vi "Write to Active Logs.vi"(7 "Async Data in":T1, 8 "error in (no error)":errorcluster, 10 "Data in":dbl[](array[numeric]), 11 "Waveform Receive in":refnum<class "Waveform Receive.lvclass">) -> (0 "error out":errorcluster, 2 "Data out":dbl[](array[numeric]), 3 "Waveform Receive out":refnum<class "Waveform Receive.lvclass">)   [LabVIEW 2015, in "Waveform Data Logger Engine.lvlib" / "Waveform Receive.lvclass"]
uses:
  Waveform Receive.lvclass
  Types/Async Data.ctl
  <vilib>/NI VeriStand/Custom Device Waveform API/Multiple Waveforms Read (DBL)/Multiple Waveforms Read (DBL).lvclass
  Utilities/Reference Dictionary/Reference Dictionary.lvclass
  Types/Wfm Acq Data.ctl
  Waveform Log/Waveform Log.lvclass
  Types/Async Communication.ctl
  Types/Check File Loop Cmd.ctl
  Waveform Receive.lvclass/Waveform Receive.ctl
  Waveform Log/Waveform Log.lvclass/Waveform Log.ctl
  Logs/Segmented Logs/Segmented Log/Segmented Log.lvclass/Segmented Log.ctl
  Shared/Classes/Log File Specifications/Log File Specification/Log File Specification.lvclass/Log File Specification.ctl
  Shared/Classes/Log File Specifications/Waveform TDMS Log File Specification/Waveform TDMS Log File Specification.lvclass/Waveform TDMS Log File Specification.ctl
  Logs/Log Files/Log File/Log File.lvclass/Log File.ctl
  Logs/Log Files/TDMS Log File/TDMS Log File.lvclass/TDMS Log File.ctl
  Logs/Log Files/Text Log File/Text Log File.lvclass/Text Log File.ctl
  Logs/Segmented Logs/Footprint Segmented Log/Footprint Segmented Log.lvclass/Footprint Segmented Log.ctl
  Logs/Segmented Logs/Time Segmented Log/Time Segmented Log.lvclass/Time Segmented Log.ctl
  Waveform Log/Get Waveform In Range.vi
  Waveform Log/Write to Waveform Log Instance.vi
  Waveform Log/Update Log Status.vi
  Logs/Segmented Logs/Segmented Log/Write Waveform to Log File Instance.vi
  Shared/Classes/Log File Specifications/Log File Specification/Get Log Specification Type.vi
  Shared/Classes/Log File Specifications/Waveform TDMS Log File Specification/Get Current Group.vi
  Logs/Log Files/Log File/Get Log File Type.vi
  Logs/Log Files/Log File/Write Channel to Log File.vi
  Logs/Log Files/TDMS Log File/Set TDMS Channel Property.vi
  Logs/Log Files/TDMS Log File/Copy Channel Properties.vi
  Logs/Segmented Logs/Segmented Log/Check Close File.vi
  Logs/Segmented Logs/Segmented Log/Check Open File.vi
  Logs/Log Files/TDMS Log File/Write Channel to TDMS Log File.vi
  Logs/Log Files/Text Log File/Write Channel to Text Log File.vi
  Logs/Segmented Logs/Segmented Log/Close Log File Instance.vi
  Logs/Segmented Logs/Segmented Log/Segment Log File.vi
  Logs/Segmented Logs/Segmented Log/Open Log File Instance.vi
  Logs/Log Files/Log File/Close Log File.vi
  Logs/Segmented Logs/Segmented Log/Make File Read-Only.vi
  Logs/Segmented Logs/Segmented Log/On Segmented Log Complete.vi
  Logs/Segmented Logs/Segmented Log/On File Close.vi
  Logs/Segmented Logs/Footprint Segmented Log/Segment Log File (Footprint).vi
  Logs/Segmented Logs/Time Segmented Log/Segment Log File (Time).vi
  Shared/Classes/Log File Specifications/Log File Specification/Open Log File.vi
  Shared/Classes/Log File Specifications/Log File Specification/Set Path Tag.vi
  Logs/Segmented Logs/Segmented Log/On File Open.vi
  Shared/Classes/Log File Specifications/Log File Specification/Set Filename Offset.vi
  Logs/Log Files/TDMS Log File/Close TDMS Log File.vi
  Logs/Log Files/Text Log File/Close Text Log File.vi
  Logs/Segmented Logs/Segmented Log/Get Current Log File Instance.vi
  Logs/Log Files/Log File/Get File Size.vi
  Logs/Log Files/Log File/Get Start Time.vi
  Shared/Classes/Log File Specifications/Log File Specification/Build File Path.vi
  Shared/Classes/Log File Specifications/Log File Specification/Resolve File Conflicts.vi
  Waveform Log/Check Instance Done.vi
  <vilib>/Utility/error.llb/Error Cluster From Error Code.vi
  Shared/Classes/Log File Specifications/Log File Specification/Initialize Log File.vi
  <vilib>/Utility/libraryn.llb/Create Directory Recursive.vi
  <vilib>/Utility/libraryn.llb/Check if File or Folder Exists.vi
  <vilib>/Utility/libraryn.llb/Get File Extension.vi
  Logs/Log Files/Text Log File/Text Log File.lvclass
  Logs/Log Files/TDMS Log File/TDMS Log File.lvclass
  Logs/Log Files/Log File/Log File.lvclass
  Logs/Segmented Logs/Time Segmented Log/Time Segmented Log.lvclass
  Logs/Segmented Logs/Footprint Segmented Log/Footprint Segmented Log.lvclass
  Shared/Classes/Log File Specifications/Waveform TDMS Log File Specification/Waveform TDMS Log File Specification.lvclass
  Waveform Data Logger Engine.lvlib
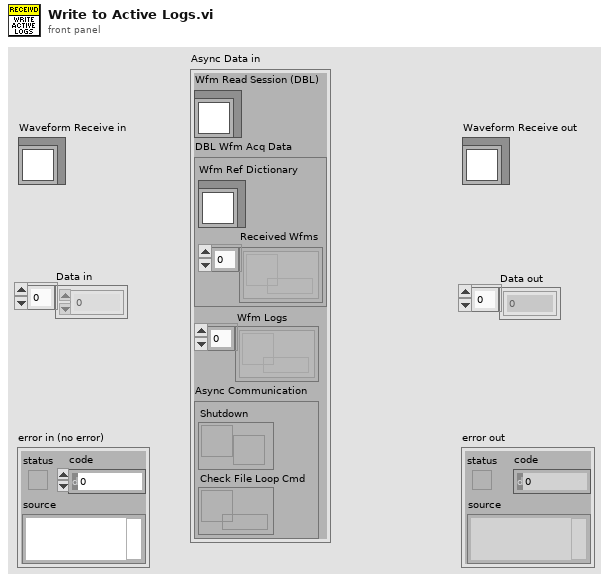
[diagram p1: front panel]
types:
  T1 = typedef "Waveform Data Logger Engine.lvlib/Async Data.ctl" = cluster{"Wfm Read Session (DBL)":refnum<class "Multiple Waveforms Read (DBL).lvclass">, "DBL Wfm Acq Data":T2, "Wfm Logs":refnum<data-value>[], "Async Communication":T3}
  T2 = typedef "Waveform Data Logger Engine.lvlib/Wfm Acq Data.ctl" = cluster{"Wfm Ref Dictionary":refnum<class "Reference Dictionary.lvclass">, "Received Wfms":refnum<data-value>[]}
  T3 = typedef "Waveform Data Logger Engine.lvlib/Async Communication.ctl" = cluster{"Shutdown":refnum<user-event>, "Check File Loop Cmd":refnum<queue>}
  T4 = typedef "Waveform Data Logger Engine.lvlib/Waveform Receive.lvclass/Associated Log.ctl" = cluster{"Log Index":i32, "Wfm Index":i32}
  T5 = typedef "Waveform Data Logger Engine.lvlib/Waveform Receive.lvclass/Wfm Info.ctl" = cluster{"Segment ID":u64, "Size":i32, "dt":dbl, "t0":timestamp, "offset":u64, "receive time":timestamp}
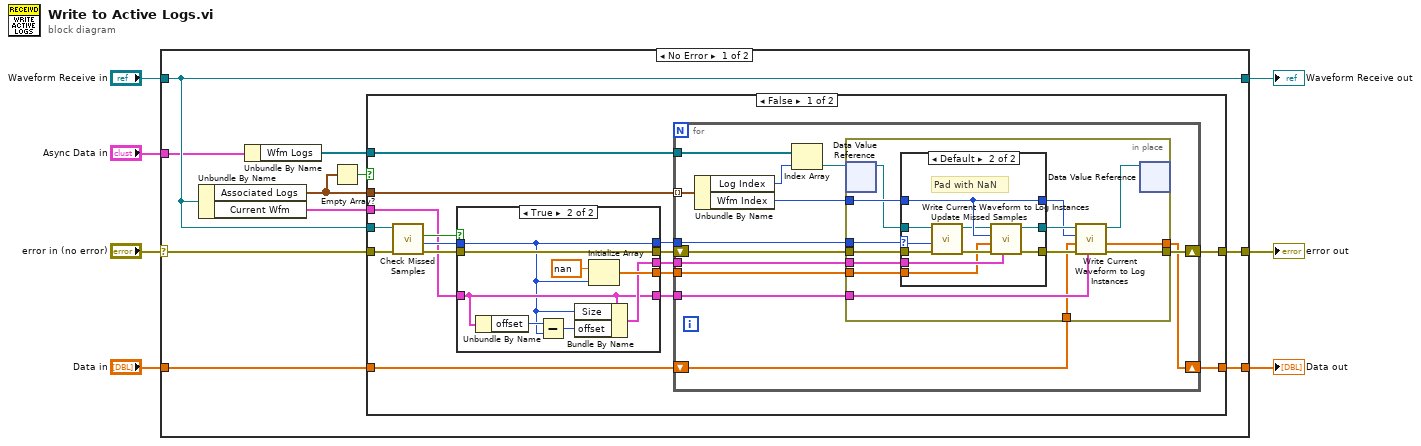
[diagram p0: block diagram]
diagram:
  n1 = case shown="No Error" "error in (no error)" {
    selector: "error in (no error)" -> [w14 w89]
    tunnel: [w16 w89] -> w6
    tunnel: [w13 w88] -> w4
    tunnel: "Waveform Receive in" -> [w13 w88]
    tunnel: "Async Data in" -> [w9 _]
    tunnel: "Data in" -> [w17 w87]
    tunnel: [w15 w87] -> w1
    frame No Error {
      n2 = Unbundle By Name(w13) -> ("Associated Logs"=w11:T4[], "Current Wfm"=w12:T5)
      n3 = Unbundle By Name(w9) -> ("Wfm Logs"=w8:refnum<data-value>[])
      n4 = Empty Array?(array=w11) -> (empty?=w10:bool)
      n5 = case shown="False" w10 {
        tunnel: w17 -> [w33 w85]
        tunnel: [w32 w86] -> w16
        tunnel: w12 -> [w20 _]
        tunnel: w11 -> [w31 _]
        tunnel: [w30 w85] -> w15
        tunnel: w14 -> [w29 w86]
        tunnel: w13 -> [w26 _]
        tunnel: w8 -> [w25 _]
        frame False {
          n6 = call "Check Missed Samples.vi"("error in (no error)"=w29, "Waveform Receive in"=w26) -> ("error out"=w21:errorcluster, "Samples Missed"=w24:u64, "Missing Samples?"=w28:bool)  [unwired: 6 in, 1 out]
          n7 = case shown="True" w28 {
            tunnel: w24 -> [w34 w37]
            tunnel: [_ w43] -> w27
            tunnel: w20 -> [w35 w38]
            tunnel: [_ w41] -> w23
            tunnel: [w36 w42] -> w22
            tunnel: w21 -> [w36 w42]
            tunnel: [w35 w38] -> w19
            tunnel: [w34 w37] -> w18
            frame False {
            }
            frame True {
              n8 = Unbundle By Name(w38) -> ("offset"=w39:u64)
              n9 = Subtract(x=w39, y=w37) -> (x-y=w40:u64)
              n10 = Bundle By Name(cluster=w38, "Size"=w37, "offset"=w40) -> (w41:T5)
              n11 = Initialize Array(nan, w37) -> (w43:dbl[])
            }
          }
          n12 = for {
            tunnel: w31 -> [w57] mode=indexing
            shift-right: [w54] -> w32
            shift-left: w22 -> [w51]
            tunnel: w25 -> [w55]
            shift-right: [w45] -> w30
            shift-left: w33 -> [w53]
            tunnel: w27 -> [w50]
            tunnel: w23 -> [w49]
            tunnel: w19 -> [w48]
            tunnel: w18 -> [w46]
            n13 = Unbundle By Name(w57) -> ("Log Index"=w56:i32, "Wfm Index"=w52:i32)
            n14 = Index Array(array=w55, index=w56) -> (element=w47:refnum<data-value>)
            n15 = in-place {
              in-place-border: [w71] -> w54
              in-place-border: w53 -> [w59]
              in-place-border: w52 -> [w68]
              in-place-border: w51 -> [w67]
              in-place-border: w50 -> [w66]
              in-place-border: w49 -> [w65]
              in-place-border: w48 -> [w60]
              in-place-border: w46 -> [w61]
              in-place-border: [w58] -> w45
              n16 = in-place-dvr #1(w47) -> (w63:refnum<class "Waveform Log.lvclass">)  [unwired: 1 out]
              n17 = case shown="Default" w61 {
                selector: w61 -> [_ w81]
                tunnel: w67 -> [w74 w83]
                tunnel: [w74 w77] -> w70
                tunnel: w68 -> [w73 w84]
                tunnel: [w72 w78] -> w69
                tunnel: w66 -> [_ w75]
                tunnel: w65 -> [_ w76]
                tunnel: [w73 w84] -> w64
                tunnel: w63 -> [w72 w82]
                frame ..0 {
                }
                frame Default {
                  # "Pad with NaN"
                  n18 = call "Update Missed Samples.vi"("error in (no error)"=w83, "Samples Missed"=w81, "Waveform Log in"=w82) -> ("error out"=w79:errorcluster, "Waveform Log out"=w80:refnum<class "Waveform Log.lvclass">)  [unwired: 7 in]
                  n19 = call "Write Current Waveform to Log Instances.vi"("Waveform Info"=w76, "error in (no error)"=w79, "Data in"=w75, "Wfm Index"=w84, "Waveform Log in"=w80) -> ("error out"=w77:errorcluster, "Waveform Log out"=w78:refnum<class "Waveform Log.lvclass">)  [unwired: 4 in, 1 out]
                }
              }
              n20 = call "Write Current Waveform to Log Instances.vi"("Waveform Info"=w60, "error in (no error)"=w70, "Data in"=w59, "Wfm Index"=w64, "Waveform Log in"=w69) -> ("error out"=w71:errorcluster, "Data out"=w58:dbl[], "Waveform Log out"=w62:refnum<class "Waveform Log.lvclass">)  [unwired: 4 in]
              n21 = in-place-dvr #1(w62) -> ()  [unwired: 2 out]
            }
          }
        }
        frame True {
        }
      }
    }
    frame Error {
    }
  }
  "error out" <- w6
  "Waveform Receive out" <- w4
  "Data out" <- w1
